vi "CascadedControl.vi"(0 "SP":T7, 1 "perturbance":sgl, 5 "PV":T6, 7 "Mode":T4, 12 "PI_Settings":T1[](array[typedef])=[{"gains"={"proportional gain"=0.0, "integral gain"=0.0}, "output range"={"output high (Inf)"=0.0, "output low (-Inf)"=0.0}, "PI_state"=enum."idle", "reset"=FALSE, "manual"=0.0}, {"gains"={"proportional gain"=0.0, "integral gain"=0.0}, "output range"={"output high (Inf)"=0.0, "output low (-Inf)"=0.0}, "PI_state"=enum."idle", "reset"=FALSE, "manual"=0.0}, {"gains"={"proportional gain"=0.0, "integral gain"=0.0}, "output range"={"output high (Inf)"=0.0, "output low (-Inf)"=0.0}, "PI_state"=enum."idle", "reset"=FALSE, "manual"=0.0}] {"gains"."proportional gain" step=0.125}) -> (4 "Vcmd":T5, 6 "Icmd":T5, 15 "Pcmd":sgl)   [LabVIEW 2017, in "ActiveFrontEnd.lvlib"]
uses:
  ActiveFrontEnd.lvlib
  CascadeControlSetpt.ctl
  CascadeControlProcVar.ctl
  DQ.ctl
  Mode.ctl
  PI_Settings.ctl
  <vilib>/rvi/Analysis/control/PID/Typedef/niFpgaPID_PIGains.ctl
  <vilib>/rvi/Analysis/control/PID/Typedef/niFpgaPID_OutputRange.ctl
  <vilib>/rvi/Analysis/control/PID/Typedef/niFpgaPID_PIState.ctl
  <vilib>/rvi/Analysis/control/PID/Typedef/niFpgaPID_ManualControl.ctl
  <userlib>/_NI FLP Library/FPGA/outsideSCTL/FlpLib Divide Shared Instance 4.vi
  <userlib>/_NI FLP Library/FPGA/outsideSCTL/FlpLib Square Shared Instance 4.vi
  <userlib>/_NI FLP Library/FPGA/outsideSCTL/FlpLib Subtract Shared Instance 4.vi
  <userlib>/_NI FLP Library/FPGA/outsideSCTL/FlpLib Square Root Shared Instance 4.vi
  <userlib>/_NI FLP Library/FPGA/outsideSCTL/FlpLib Multiply Shared Instance 4.vi
  <userlib>/_NI FLP Library/FPGA/outsideSCTL/FlpLib Negate Outside SCTL.vi
  <userlib>/_NI FLP Library/FPGA/outsideSCTL/FlpLib Multiply Shared Instance 3.vi
  <userlib>/_NI FLP Library/addons/Control/PI_Controller/FlpLib PI_Controller 4.vi
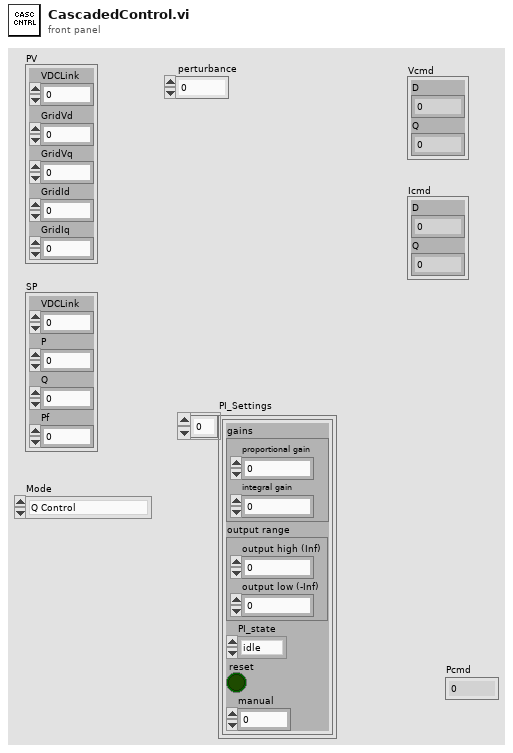
[diagram p1: front panel]
types:
  T1 = typedef "ActiveFrontEnd.lvlib/PI_Settings.ctl" = cluster{"gains":T2, "output range":T3, "PI_state":enum8{"idle", "normal", "manual", "perturbance"}, "reset":bool, "manual":sgl}
  T2 = typedef "niFpgaPID_PIGains.ctl" = cluster{"proportional gain":sgl, "integral gain":sgl}
  T3 = typedef "niFpgaPID_OutputRange.ctl" = cluster{"output high (Inf)":sgl, "output low (-Inf)":sgl}
  T4 = typedef "ActiveFrontEnd.lvlib/Mode.ctl" = enum16{"Q Control", "Pf Control"}
  T5 = typedef "ActiveFrontEnd.lvlib/DQ.ctl" = cluster{"D":sgl, "Q":sgl}
  T6 = typedef "ActiveFrontEnd.lvlib/CascadeControlProcVar.ctl" = cluster{"VDCLink":sgl, "GridVd":sgl, "GridVq":sgl, "GridId":sgl, "GridIq":sgl}
  T7 = typedef "ActiveFrontEnd.lvlib/CascadeControlSetpt.ctl" = cluster{"VDCLink":sgl, "P":sgl, "Q":sgl, "Pf":sgl}
  T8 = typedef "niFpgaPID_PIState.ctl" = cluster{"uI(k-1)":sgl, "e(k-1)":sgl, "output (k-1)":sgl}
  T9 = typedef "niFpgaPID_ManualControl.ctl" = cluster{"manual? (F)":bool, "manual input (0)":sgl}
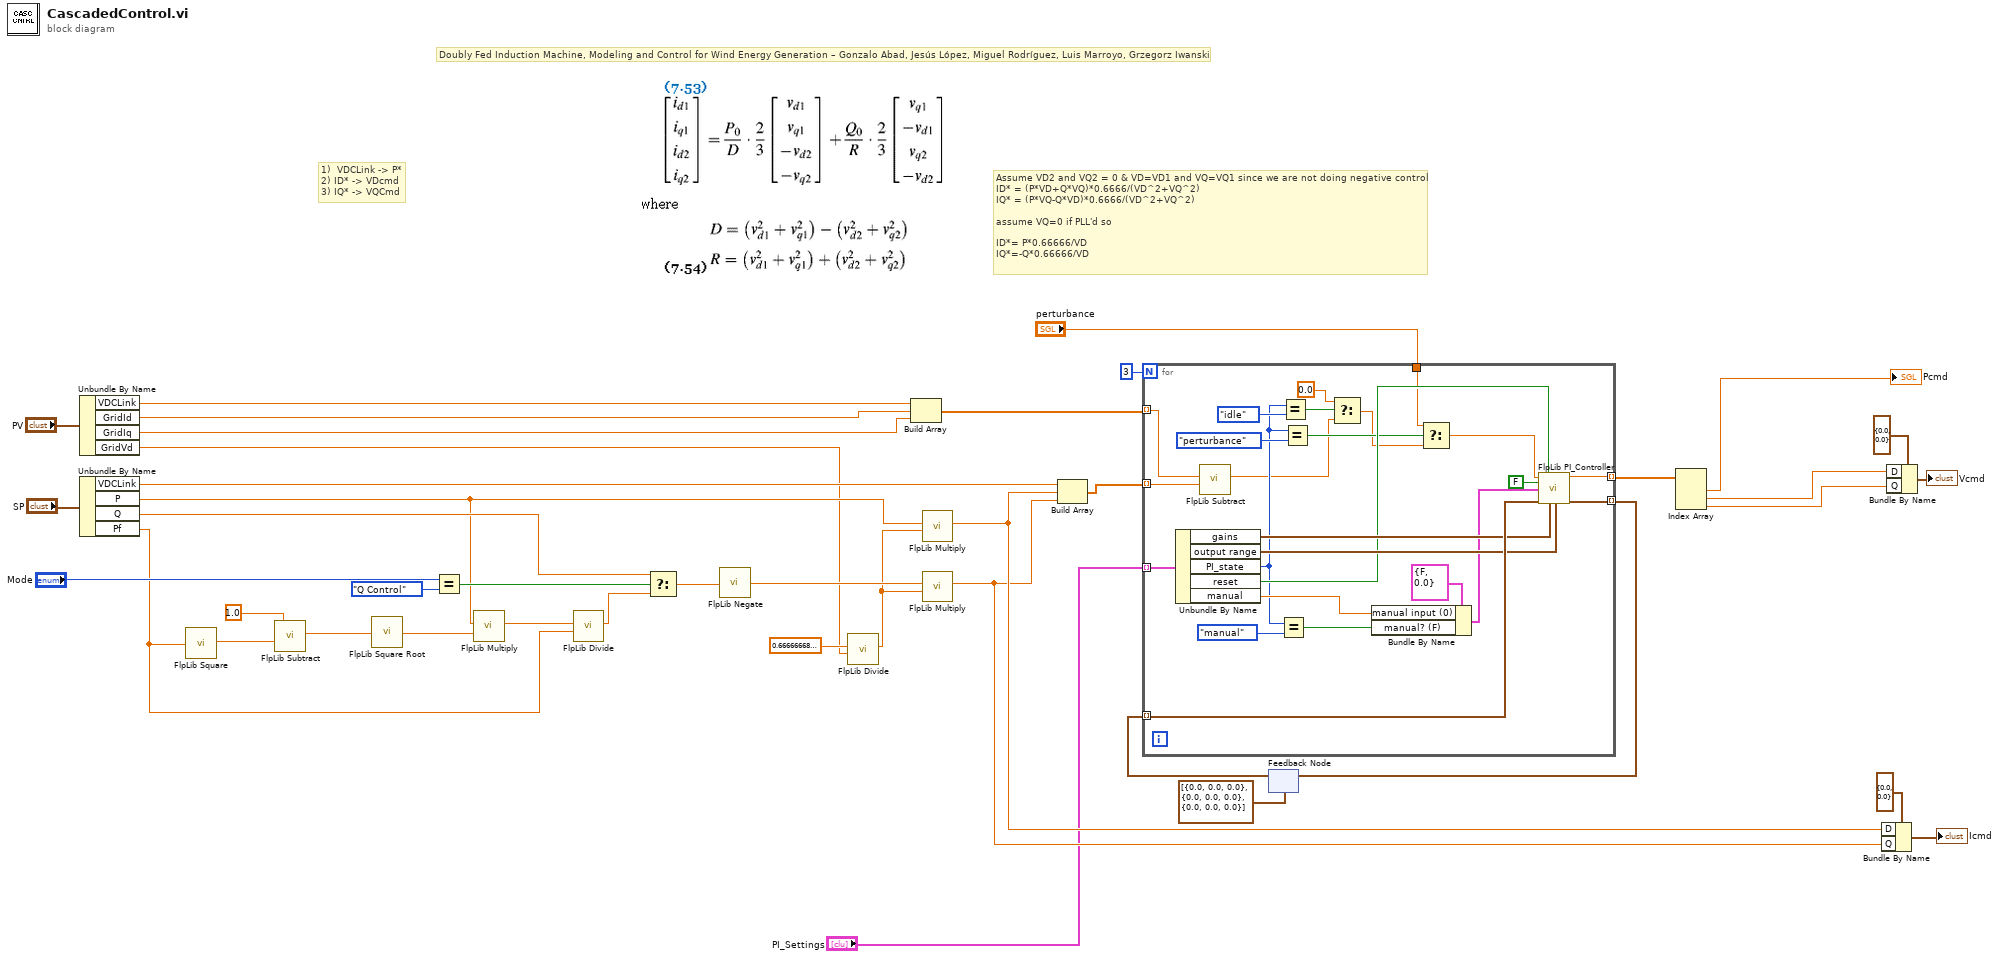
[diagram p0: block diagram]
diagram:
  # "Assume VD2 and VQ2 = 0 & VD=VD1 and VQ=VQ1 since we are not doing negative control\nID* = (P*VD+Q*VQ)*0.6666/(VD^2+VQ^2)\nIQ* = (P*VQ-Q*VD)*0.6666/(VD^2+VQ^2)\n\nassume VQ=0 if PLL'd so\n\nID*= P*0.66666/VD\nIQ*=-Q*0.66666/VD"
  # "Doubly Fed Induction Machine, Modeling and Control for Wind Energy Generation – Gonzalo Abad, Jesús López, Miguel Rodríguez, Luis Marroyo, Grzegorz Iwanski"
  # "1)  VDCLink -> P*\n2) ID* -> VDcmd\n3) IQ* -> VQCmd"
  n1 = Unbundle By Name("PV") -> ("VDCLink"=w17:sgl, "GridId"=w16:sgl, "GridIq"=w15:sgl, "GridVd"=w3:sgl)
  n2 = Unbundle By Name("SP") -> ("VDCLink"=w19:sgl, "P"=w25:sgl, "Q"=w30:sgl, "Pf"=w23:sgl)
  n3 = call-poly <userlib>:"FlpLib Square.vi"("x"=w23) -> ("x^2"=w29:sgl)  [unwired: 4 in]
  n4 = call-poly <userlib>:"FlpLib Subtract.vi"("y"=w29, "x"=sgl 1.0) -> ("x-y"=w27:sgl)  [unwired: 5 in]
  n5 = call-poly <userlib>:"FlpLib Square Root.vi"("x"=w27) -> ("sqrt(x)"=w26:sgl)  [unwired: 4 in]
  n6 = Equal?(x="Mode", y=Mode."Q Control") -> (x = y?=w31:bool)
  n7 = call-poly <userlib>:"FlpLib Multiply.vi"("y"=w26, "x"=w25) -> ("x*y"=w24:sgl)  [unwired: 5 in]
  n8 = call-poly <userlib>:"FlpLib Divide.vi"("y"=w23, "x"=w24) -> ("x/y"=w22:sgl)  [unwired: 5 in]
  n9 = Select(t=w30, s=w31, f=w22) -> (s? t:f=w21:sgl)
  n10 = call-poly <userlib>:"FlpLib Negate.vi"("x"=w21) -> ("-x"=w20:sgl)  [unwired: 4 in]
  n11 = call-poly <userlib>:"FlpLib Divide.vi"("y"=w3, "x"=sgl 0.6666667) -> ("x/y"=w1:sgl)  [unwired: 5 in]
  n12 = Build Array(w17, w16, w15) -> (w14:sgl[])
  n13 = call-poly <userlib>:"FlpLib Multiply.vi"("y"=w1, "x"=w25) -> ("x*y"=w13:sgl)  [unwired: 5 in]
  n14 = call-poly <userlib>:"FlpLib Multiply.vi"("y"=w1, "x"=w20) -> ("x*y"=w12:sgl)  [unwired: 5 in]
  n15 = Build Array(w19, w13, w12) -> (w18:sgl[])
  n16 = feedback #1(T8[] [{"uI(k-1)"=0.0, "e(k-1)"=0.0, "output (k-1)"=0.0}, {"uI(k-1)"=0.0, "e(k-1)"=0.0, "output (k-1)"=0.0}, {"uI(k-1)"=0.0, "e(k-1)"=0.0, "output (k-1)"=0.0}]) -> (w5:T8[])
  n17 = for {
    N: 3 -> [_]
    tunnel: w14 -> [w65] mode=indexing
    tunnel: w18 -> [w66] mode=indexing
    tunnel: [w64] -> w11 mode=indexing
    tunnel: [w63] -> w7 mode=indexing
    tunnel: w5 -> [w62] mode=indexing
    tunnel: "PI_Settings" -> [w61] mode=indexing
    tunnel: "perturbance" -> [w43]
    n18 = Unbundle By Name(w61) -> ("gains"=w60:T2, "output range"=w59:T3, "PI_state"=w49:enum8{"idle", "normal", "manual", "perturbance"}, "reset"=w51:bool, "manual"=w52:sgl)
    n19 = call-poly <userlib>:"FlpLib Subtract.vi"("y"=w66, "x"=w65) -> ("x-y"=w45:sgl)  [unwired: 5 in]
    n20 = Equal?(x=w49, y=enum8{"idle", "normal", "manual", "perturbance"}."manual") -> (x = y?=w53:bool)
    n21 = Equal?(x=w49, y=enum8{"idle", "normal", "manual", "perturbance"}."idle") -> (x = y?=w48:bool)
    n22 = Equal?(x=w49, y=enum8{"idle", "normal", "manual", "perturbance"}."perturbance") -> (x = y?=w47:bool)
    n23 = Select(t=sgl 0.0, s=w48, f=w45) -> (s? t:f=w44:sgl)
    n24 = Bundle By Name(cluster=T9 {"manual? (F)"=FALSE, "manual input (0)"=0.0} ("manual control"), "manual input (0)"=w52, "manual? (F)"=w53) -> (w54:T9)
    n25 = Select(t=w43, s=w47, f=w44) -> (s? t:f=w42:sgl)
    n26 = call-poly <userlib>:"FlpLib PI_Controller.vi"("error"=w42, "reset? (F)"=w51, "enable bumpless transfer? (F)"=FALSE, "manual control"=w54, "state in"=w62, "gains"=w60, "output range"=w59) -> ("output"=w64:sgl, "state out"=w63:T8)  [unwired: 5 in, 2 out]
  }
  n27 = feedback-in #1(w7) -> ()
  n28 = Index Array(array=w11) -> (element #1=→"Pcmd":sgl, element #2=w10:sgl, element #3=w9:sgl)  [unwired: 3 in]
  n29 = Bundle By Name(cluster=T5 {"D"=0.0, "Q"=0.0} ("DQ"), "D"=w13, "Q"=w12) -> (→"Icmd":T5)
  n30 = Bundle By Name(cluster=T5 {"D"=0.0, "Q"=0.0} ("DQ"), "D"=w10, "Q"=w9) -> (→"Vcmd":T5)
